vi "New Rotation State.vi"(10 "Move":T2, 11 "Rotation State":T1) -> (3 "New Rotation State":T1)   [LabVIEW 2017]
uses:
  Controls/Moves.ctl
  Controls/Rotation State.ctl
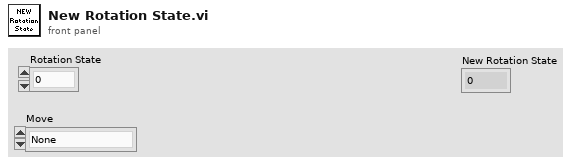
[diagram p1: front panel]
types:
  T1 = typedef "Rotation State.ctl" = enum16{"0", "90", "180", "270"}
  T2 = typedef "Moves.ctl" = enum16{"None", "Right", "Left", "Step Down", "Go Down", "90 Clockwise", "90 Anti-Clockwise"}
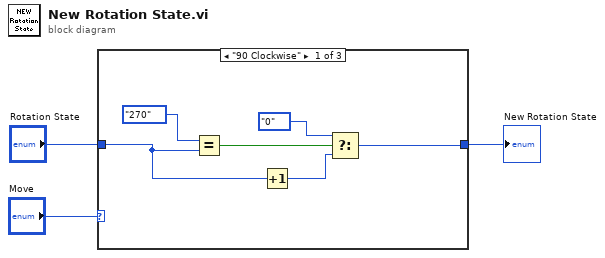
[diagram p0: block diagram]
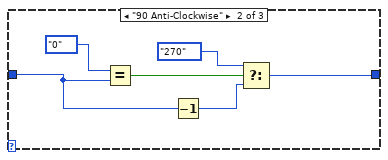
[diagram p2: hidden frame]
diagram:
  n1 = case shown="\"90 Clockwise\"" "Move" {
    tunnel: "Rotation State" -> [w6 w12 w16]
    tunnel: [w7 w13 w16] -> w1
    frame "90 Clockwise" {
      n2 = Equal?(x=Rotation_State."270" ("y"), y=w6) -> (x = y?=w8:bool)
      n3 = Increment(x=w6) -> (x+1=w5:T1)
      n4 = Select(t=Rotation_State."0" ("cas vrai"), s=w8, f=w5) -> (s? t:f=w7:T1)
    }
    frame "90 Anti-Clockwise" {
      n5 = Equal?(x=Rotation_State."0" ("y"), y=w12) -> (x = y?=w14:bool)
      n6 = Decrement(x=w12) -> (x-1=w11:T1)
      n7 = Select(t=Rotation_State."270" ("cas vrai"), s=w14, f=w11) -> (s? t:f=w13:T1)
    }
    frame Default {
    }
  }
  "New Rotation State" <- w1
